vi "Big Endian.vi"() -> (0 "big endian":bool)   [LabVIEW 2017]
panel:
  # "LVHDF5 Toolkit\nCopyright (c) 2005-2013 by Jason D. Sommerville\nCopyright (c) 2014 by UPVI, LLC.\n\nThis use and distribution of this file is governed by the terms found in \nLICENSE.txt distributed with this toolkit and installed at\n <user.lib>\\_lvhdf5\\LICENSE.txt"
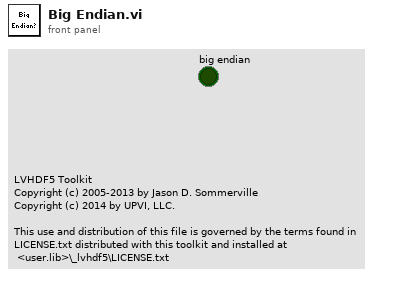
[diagram p1: front panel]
types:
  T1 = enum16{"big-endian, network order", "native, host order", "little-endian"}
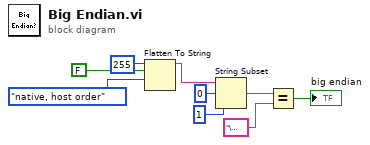
[diagram p0: block diagram]
diagram:
  n1 = Flatten To String(anything=255, prepend array or string size? (T)=FALSE, byte order (0:big-endian, network order)=T1."native, host order") -> (data string=w6:string)  [unwired: 1 in, 2 out]
  n2 = String Subset(string=w6, offset (0)=0, length (rest)=1 ("length (rest)")) -> (substring=w2:string)
  n3 = Equal?(x=w2, y="\u0000" ("x")) -> (x = y?=→"big endian":bool)
